vi "Read Measurement Data (Analog 1Chan).vi"(0 "VISA resource name":refnum<visa-resource-name>, 5 "Channel (0001)":string="0001", 9 "Data Format (0 : Binary)":i32(ring) items=["Binary", "ASCII"], 11 "error in (no error)":errorcluster) -> (2 "Date Time":timestamp=timestamp(3345116400 s since 1904-01-01) format="%<%H:%M:%S%3u\n%x>T", 4 "VISA resource name out":refnum<visa-resource-name>, 6 "Channel":string, 8 "Data":dbl format="%.4f", 10 "Data Status":i32(ring) items=["Normal", "Differential Input", "Skip", "Over", "Error", "Burnout", "Power Failure"], 13 "Alarm Status":i32[](array[ring]) items=["No Alarm", "High Limit Alarm (H)", "Low Limit Alarm (L)", "Difference High Limit Alarm (h)", "Difference Low Limit Alarm (l)", "High Limit on Rate-of-change Alarm (R)", "Low Limit on Rate-of-change Alarm (r)", "Delay High Limit Alarm (T)", "Delay Low Limit Alarm (t)"], 14 "Unit":string, 15 "error out":errorcluster)   [LabVIEW 2020, in "Yokogawa GX Series.lvlib"]
doc: "This VI reads the analog measurement data by ASCII or Binary."
uses:
  <instrlib>/Yokogawa GX Series/Yokogawa GX Series.lvlib
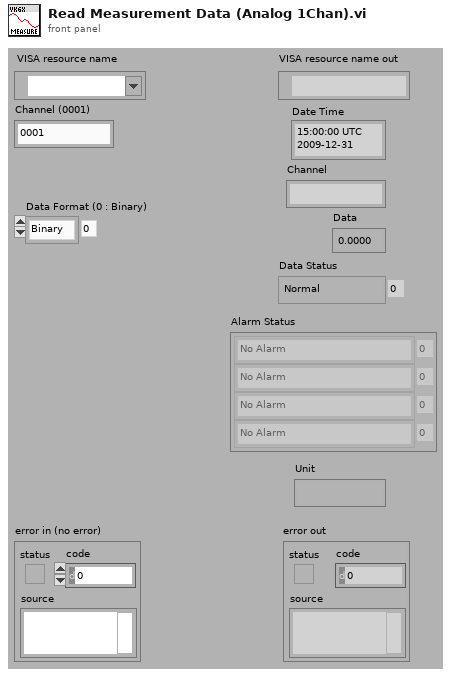
[diagram p1: front panel]
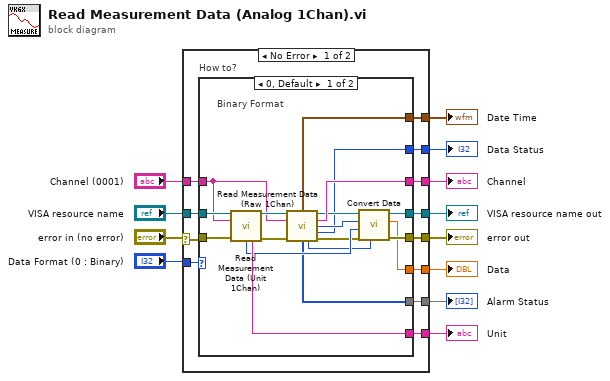
[diagram p0: block diagram]
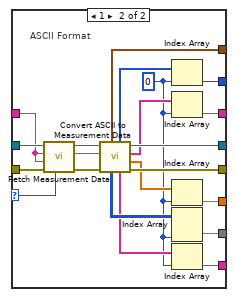
[diagram p2: hidden frame]
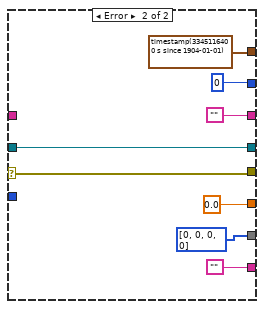
[diagram p3: hidden frame]
diagram:
  n1 = case shown="No Error" "error in (no error)" {
    selector: "error in (no error)" -> [w13 w70]
    tunnel: "VISA resource name" -> [w24 w71]
    tunnel: [w23 w71] -> w11
    tunnel: [w22 w70] -> w10
    tunnel: "Data Format (0 : Binary)" -> [w21 _]
    tunnel: [w20 ""] -> w8
    tunnel: [w19 timestamp(3345116400 s since 1904-01-01)] -> w7
    tunnel: [w18 ""] -> w6
    tunnel: [w17 0.0] -> w5
    tunnel: [w16 i32[] [0, 0, 0, 0]] -> w4
    tunnel: [w15 0] -> w3
    tunnel: "Channel (0001)" -> [w14 _]
    frame No Error {
      n2 = case "How to?" shown="0, Default" w21 {
        selector: w21 -> [_ w43]
        tunnel: w24 -> [w40 w63]
        tunnel: w13 -> [w39 w62]
        tunnel: [w42 w57] -> w23
        tunnel: [w41 w59] -> w22
        tunnel: w14 -> [w26 w46]
        tunnel: [w37 w47] -> w20
        tunnel: [w33 w58] -> w19
        tunnel: [w32 w53] -> w18
        tunnel: [w38 w52] -> w17
        tunnel: [w27 w51] -> w15
        tunnel: [w30 w50] -> w16
        frame 0, Default {
          # "Binary Format"
          n3 = call <instrlib>:"Read Measurement Data (Unit 1Chan).vi"("VISA resource name"=w40, "Channel (1)"=w26, "error in (no error)"=w39) -> ("VISA resource name out"=w35:refnum<visa-resource-name>, "Decimal Position"=w36:i32, "Unit"=w37:string, "error out"=w34:errorcluster)  [unwired: 9 out]
          n4 = call <instrlib>:"Read Measurement Data (Raw 1Chan).vi"("VISA resource name"=w35, "Channel (1)"=w26, "error in (no error)"=w34) -> ("Date Time"=w33:timestamp, "VISA resource name out"=w28:refnum<visa-resource-name>, "Channel"=w32:string, "Data"=w31:i32, "Data Status"=w27:i32, "Alarm Status"=w30:i32[], "Data Type"=w25:i32, "error out"=w29:errorcluster)  [unwired: 5 out]
          n5 = call <instrlib>:"Convert Data.vi"("Data Type (1 : Int)"=w25, "error in (no error)"=w29, "Decimal Position (0)"=w36, "Integer Data (0)"=w31, "VISA resource name"=w28) -> ("error out"=w41:errorcluster, "Float Data"=w38:dbl, "VISA resource name out"=w42:refnum<visa-resource-name>)  [unwired: 4 out]
        }
        frame 1 {
          w44 = 0
          # "ASCII Format"
          n6 = call <instrlib>:"Fetch Measurement Data.vi"("Data Format (0 : Binary)"=w43, "error in (no error)"=w62, "End Channel (1)"=w46, "Start Channel (1)"=w46, "VISA resource name"=w63) -> ("error out"=w60:errorcluster, "Measurement Data"=w45:string, "VISA resource name out"=w61:refnum<visa-resource-name>)  [unwired: 4 out]
          n7 = call <instrlib>:"Convert ASCII to Measurement Data.vi"("error in (no error)"=w60, "Measurement ASCII Data (\"\")"=w45, "VISA resource name"=w61) -> ("error out"=w59:errorcluster, "Data"=w55:dbl[], "Channel"=w56:string[], "VISA resource name out"=w57:refnum<visa-resource-name>, "Unit"=w48:string[], "Data Status"=w54:i32[], "Alarm Status"=w49:i32[][], "Date Time"=w58:timestamp)  [unwired: 1 in]
          n8 = Index Array(array=w54, index=w44) -> (element=w51:i32)
          n9 = Index Array(array=w56, index=w44) -> (element=w53:string)
          n10 = Index Array(array=w55, index=w44) -> (element=w52:dbl)
          n11 = Index Array(array=w49, index (col)=w44) -> (element=w50:i32[])  [unwired: 1 in]
          n12 = Index Array(array=w48, index=w44) -> (element=w47:string)
        }
      }
    }
    frame Error {
    }
  }
  "error out" <- w10
  "VISA resource name out" <- w11
  "Unit" <- w8
  "Channel" <- w6
  "Alarm Status" <- w4
  "Date Time" <- w7
  "Data" <- w5
  "Data Status" <- w3
